vi "Read sensor to DB.vi"() -> ()   [LabVIEW 2018]
panel:
  in  "Temperature Mode":string(combo)="Software PID"
  out "Waveform Chart":dbl(graph)
  in  "SampleTme [sec]":dbl
  in  "Stop":bool
  out "Thermometer":dbl(slide) scale=0.0..100.0
  in  "Temp unit":enum16{"Celsius", "Fahrenheit"}(ring)
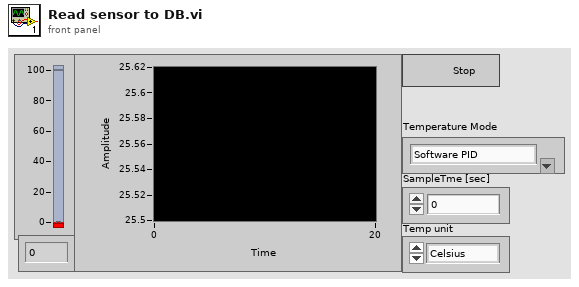
[diagram p1: front panel]
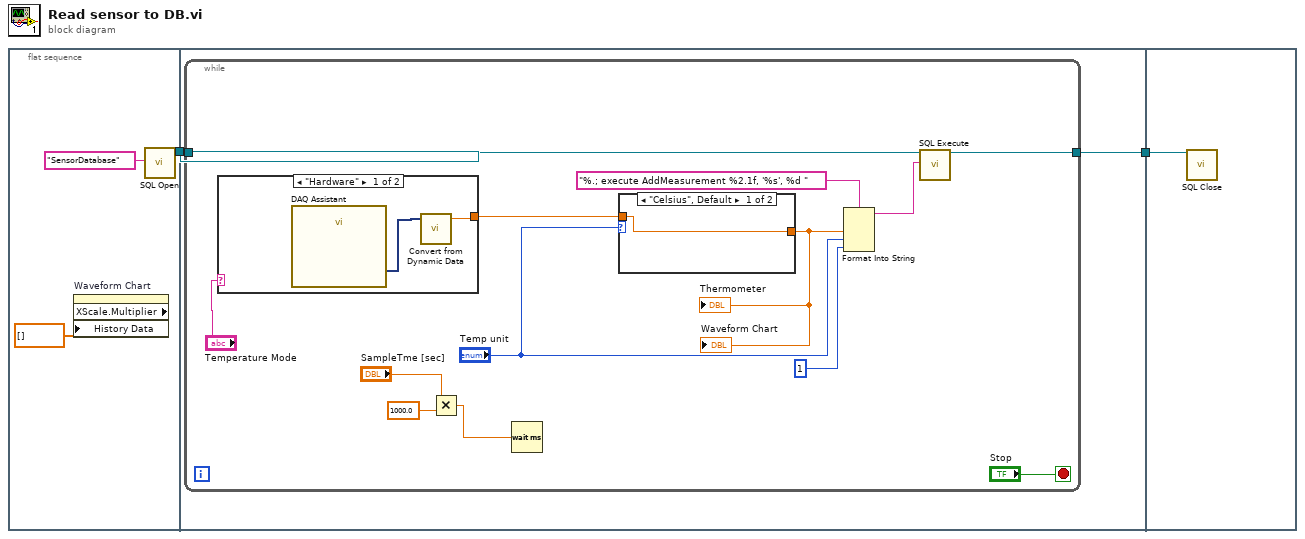
[diagram p0: block diagram]
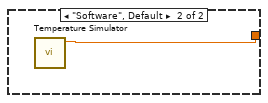
[diagram p2: hidden frame]
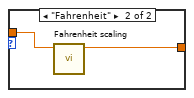
[diagram p3: hidden frame]
diagram:
  n1 = flat-sequence {
    tunnel: [w5] -> w2
    tunnel: w2 -> [w7]
    tunnel: [w6] -> w1
    tunnel: w1 -> [w27]
    frame #0 {
      n2 = property on="Waveform Chart" class="WFChart (strict)" props=["XScale", "Multiplier", "History Data"]("History Data"=dbl[] []) -> ()  [unwired: 2 in, 3 out]
      n3 = call <vilib>:"SQL Open.vi"("ConnectionString In"="SensorDatabase") -> ("Connection Out"=w5:refnum<k7>)  [unwired: 17 in, 1 out]
    }
    frame #1 {
      n4 = while {
        tunnel: w7 -> [w19]
        tunnel: [w18] -> w6
        stop <- "Stop" stop-if-true
        n5 = case shown="\"Hardware\"" "Temperature Mode" {
          tunnel: [w21 w23] -> w8
          frame "Hardware" {
            n6 = call "DAQ Assistant"() -> ("data"=w22:dynamicdata)  [unwired: 17 in, 2 out]
            n7 = call "Convert from Dynamic Data"("Dynamic Data Type"=w22) -> ("Scalar"=w21:dbl)  [unwired: 3 in]
          }
          frame "Software", Default {
            n8 = call "Temperature Simulator.vi"() -> ("Temperature Value"=w23:dbl)  [unwired: 11 in]
          }
        }
        n9 = Multiply(x="SampleTme [sec]", y=1000.0) -> (x*y=w12:dbl)
        n10 = Wait (ms)(milliseconds to wait=w12) -> ()  [unwired: 1 out]
        n11 = case shown="\"Celsius\", Default" "Temp unit" {
          tunnel: [w24 w26] -> w10
          tunnel: w8 -> [w24 w25]
          frame "Celsius", Default {
          }
          frame "Fahrenheit" {
            n12 = call "Fahrenheit scaling.vi"("Tc"=w25) -> ("Tf"=w26:dbl)  [unwired: 10 in]
          }
        }
        "Thermometer" <- w10
        "Waveform Chart" <- w10
        n13 = Format Into String(format string="%.; execute AddMeasurement %2.1f, '%s', %d ", w10, "Temp unit", u32 1 ("milliseconds to wait")) -> (resulting string=w17:string)  [unwired: 2 in, 1 out]
        n14 = call <vilib>:"SQL Execute.vi"("Connection In"=w19, "SQL Query"=w17) -> ("Connection Out"=w18:refnum<k7>)  [unwired: 16 in, 1 out]
      }
    }
    frame #2 {
      n15 = call <vilib>:"SQL Close.vi"("Connection In"=w27) -> ()  [unwired: 18 in, 1 out]
    }
  }
